vi "continuous mag sensor.vi"() -> ()   [LabVIEW 2012]
doc: "This example demonstrates how to continuously acquire buffered voltage measurements using a DAQmx device.\n\nFor instructions on how to connect your signals to the DAQ device, refer to your device documentation."
uses:
  <vilib>/DAQmx/write.llb/DAQmx Write (Analog DBL 1Chan 1Samp).vi
  <vilib>/DAQmx/read.llb/DAQmx Read (Analog 1D Wfm NChan NSamp).vi
  <vilib>/DAQmx/create/channels.llb/DAQmx Create Channel (AI-Voltage-Basic).vi
  <vilib>/DAQmx/configure/timing.llb/DAQmx Timing (Sample Clock).vi
  <vilib>/DAQmx/create/channels.llb/DAQmx Create Channel (AO-Voltage-Basic).vi
  <vilib>/DAQmx/miscellaneous.llb/DAQmx Fill In Error Info.vi
panel:
  in  "output voltage":dbl format="%0.2f"
  in  "Stop":bool
  out "Waveform Graph":waveform(dbl)[](graph)
  in  "Samples per Loop":i32=1000
  in  "Sample Rate":dbl=1000.0
  in  "Sample Clock Source":tag="OnboardClock"
  in  "Terminal Configuration":i32(ring)=-1 items=["default"=-1, "RSE"=10083, "NRSE"=10078, "Differential"=10106, "Pseudodifferential"=12529]
  in  "Max Voltage":dbl=5.0
  in  "Min Voltage":dbl=-5.0
  # "Channel Settings"
  # "Acquired Data"
  # "Timing Settings"
  # "Logging Settings"
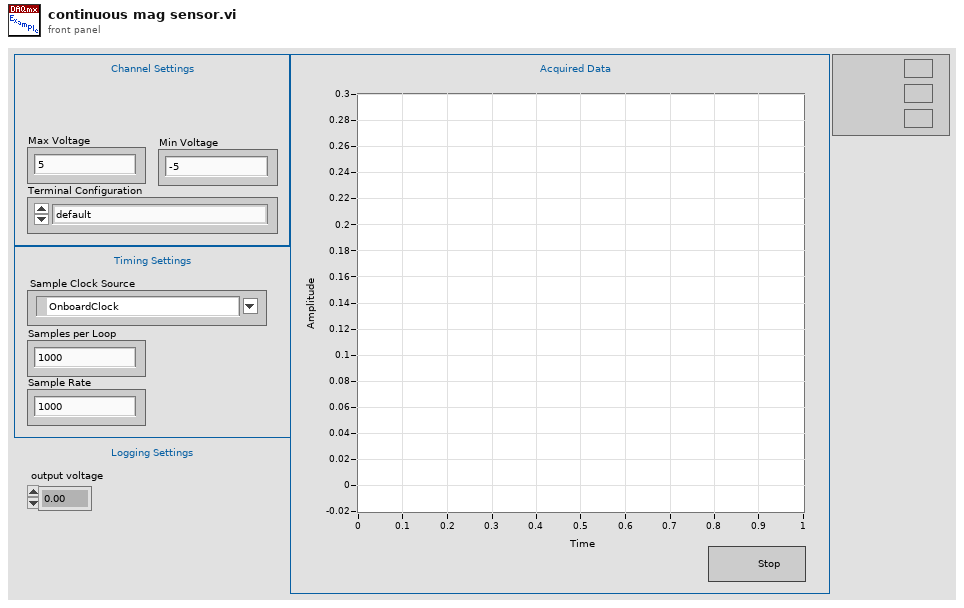
[diagram p1: front panel]
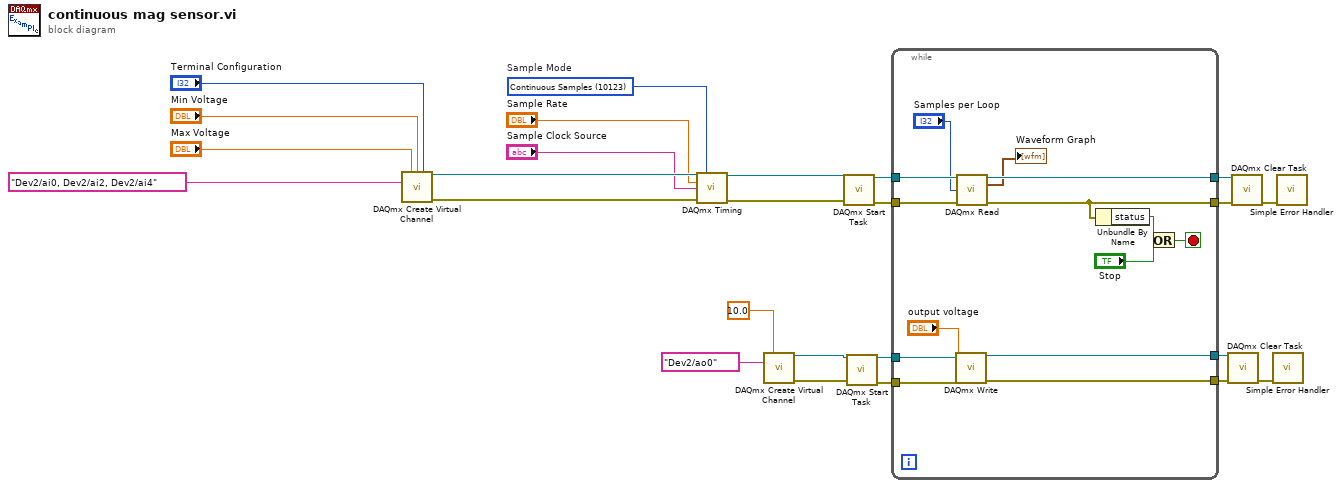
[diagram p0: block diagram]
diagram:
  w25 = 10123 items=["Finite Samples"=10178, "Continuous Samples"=10123, "Hardware Timed Single Point"=12522]  # Sample Mode
  n1 = call-poly <vilib>:"DAQmx Create Virtual Channel.vi"("maximum value"="Max Voltage", "minimum value"="Min Voltage", "input terminal configuration"="Terminal Configuration", "physical channels"=tag "Dev2/ai0, Dev2/ai2, Dev2/ai4" ("Physical Channel")) -> ("task out"=w16:refnum<k21>, "error out"=w15:errorcluster)  [unwired: 10 in]
  n2 = call-poly <vilib>:"DAQmx Timing.vi"("task/channels in"=w16, "sample mode"=w25, "rate"="Sample Rate", "source"="Sample Clock Source", "error in"=w15) -> ("task out"=w14:refnum<k21>, "error out"=w13:errorcluster)  [unwired: 9 in]
  n3 = call-poly <vilib>:"DAQmx Create Virtual Channel.vi"("maximum value"=10.0, "physical channels"=tag "Dev2/ao0") -> ("task out"=w2:refnum<k21>, "error out"=w1:errorcluster)  [unwired: 12 in]
  n4 = call <vilib>:"DAQmx Start Task.vi"("task/channels in"=w14, "error in"=w13) -> ("task out"=w24:refnum<k21>, "error out"=w23:errorcluster)  [unwired: 12 in]
  n5 = call <vilib>:"DAQmx Start Task.vi"("task/channels in"=w2, "error in"=w1) -> ("task out"=w9:refnum<k21>, "error out"=w8:errorcluster)  [unwired: 12 in]
  n6 = while {
    tunnel: w24 -> [w39]
    tunnel: w23 -> [w38]
    tunnel: [w35] -> w21
    tunnel: [w36] -> w22
    tunnel: w9 -> [w30]
    tunnel: w8 -> [w29]
    tunnel: [w27] -> w6
    tunnel: [w26] -> w5
    stop <- w37 stop-if-true
    n7 = call-poly <vilib>:"DAQmx Write.vi"("task/channels in"=w30, "data"="output voltage", "error in"=w29) -> ("task out"=w27:refnum<k21>, "error out"=w26:errorcluster)  [unwired: 10 in, 1 out]
    n8 = call-poly <vilib>:"DAQmx Read.vi"("task/channels in"=w39, "number of samples per channel"="Samples per Loop", "error in"=w38) -> ("task out"=w36:refnum<k21>, "data"=→"Waveform Graph":waveform(dbl)[], "error out"=w35:errorcluster)  [unwired: 10 in]
    n9 = Unbundle By Name(w35) -> ("status"=w34:bool)
    n10 = Or(x=w34, y="Stop") -> (x .or. y?=w37:bool)
  }
  n11 = call <vilib>:"DAQmx Clear Task.vi"("task in"=w6, "error in"=w5) -> ("error out"=w7:errorcluster)  [unwired: 13 in]
  n12 = call <vilib>:"DAQmx Clear Task.vi"("task in"=w22, "error in"=w21) -> ("error out"=w20:errorcluster)  [unwired: 13 in]
  n13 = call <vilib>:"Simple Error Handler.vi"("error in (no error)"=w7) -> ()  [unwired: 4 in, 5 out]
  n14 = call <vilib>:"Simple Error Handler.vi"("error in (no error)"=w20) -> ()  [unwired: 4 in, 5 out]
